vi "CoolProp_SI_V15.0.vi"(4 "Value2":dbl=1.0, 5 "Value1":dbl=400.0, 6 "Input Variable #2":T1(ring), 7 "Input Variable #1":T2(ring), 8 "error in (no error)":errorcluster, 9 "Output":string="H", 10 "Fluid":string="Water", 11 "path in":path=path "C:/Program Files (x86)/National Instruments/LabVIEW 2015/user.lib/CoolProp.dll") -> (0 "error out":errorcluster, 2 "error_message":string, 3 "Return Value":dbl=416.75835925510785)   [LabVIEW 2015]
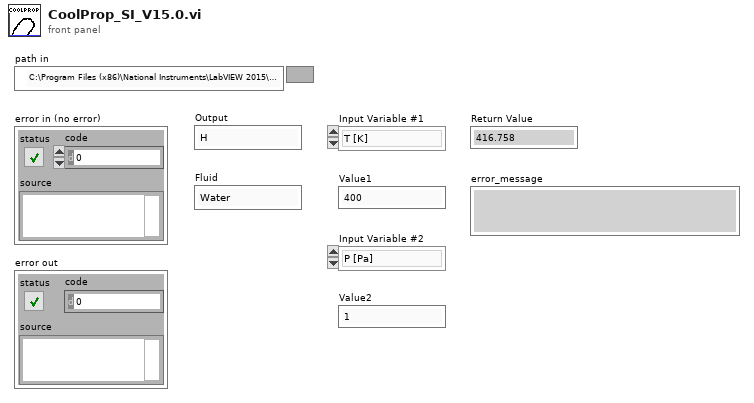
[diagram p1: front panel]
types:
  T1 = enum16{"P [Pa]", "D [kg/m3]", "Q [–]", "H [J/kg]", "S [J/kg-K]"}
  T2 = enum16{"T [K]", "P [Pa]", "H [J/kg]", "S [J/kg-K]"}
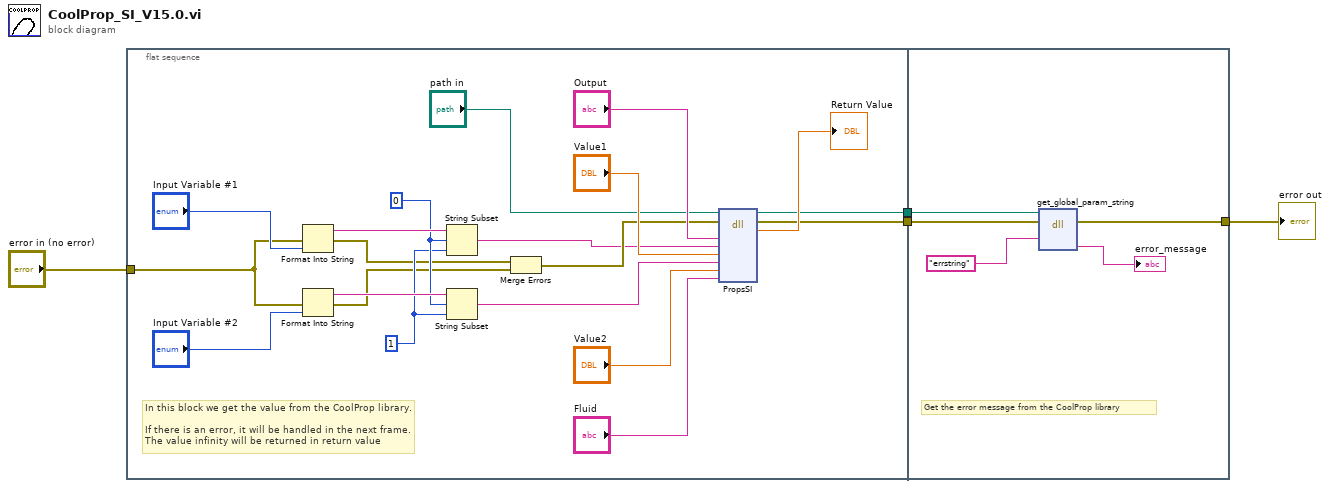
[diagram p0: block diagram]
diagram:
  n1 = flat-sequence {
    tunnel: "error in (no error)" -> [w8]
    tunnel: [w7] -> w3
    tunnel: [w6] -> w1
    tunnel: w3 -> [w27]
    tunnel: [w26] -> w2
    tunnel: w1 -> [w25]
    frame #0 {
      w16 = 1 ("length (rest)")
      w17 = 0 ("offset (0)")
      # "In this block we get the value from the CoolProp library.\n\nIf there is an error, it will be handled in the next frame.\nThe value infinity will be returned in return value"
      n2 = Format Into String(error in=w8, "Input Variable #1") -> (resulting string=w19:string, error out=w15:errorcluster)  [unwired: 2 in]
      n3 = Format Into String(error in=w8, "Input Variable #2") -> (resulting string=w18:string, error out=w14:errorcluster)  [unwired: 2 in]
      n4 = String Subset(string=w19, offset (0)=w17, length (rest)=w16) -> (substring=w10:string)
      n5 = String Subset(string=w18, offset (0)=w17, length (rest)=w16) -> (substring=w9:string)
      n6 = Merge Errors(w15, w14) -> (w13:errorcluster)
      n7 = dll-call lib="C:/Program Files (x86)/National Instruments/LabVIEW 2015/user.lib/CoolProp.dll" fn="PropsSI"(path in="path in", error in=w13, "Output"="Output", "Input1"=w10, "Value1"="Value1", "Input2"=w9, "Value2"="Value2", "Fluid"="Fluid") -> (path out=w6:path, error out=w7:errorcluster, "OutputValue"=→"Return Value":dbl)  [unwired: 7 in]
    }
    frame #1 {
      # "Get the error message from the CoolProp library"
      n8 = dll-call lib="C:/Program Files (x86)/National Instruments/LabVIEW 2011/user.lib/CoolProp.dll" fn="get_global_param_string"(path in=w25, error in=w27, "param"="errstring") -> (error out=w26:errorcluster, "error_message"=→"error_message":string)  [unwired: 2 in, 3 out]
    }
  }
  "error out" <- w2
